vi "main.vi"() -> ()   [LabVIEW 2021]
uses:
  <vilib>/addons/Sound and Vibration/svt_Controls/subVIs/SV Intensity Graph.ctl
  <vilib>/sound2/lvsound2.llb/Sound Data Format.ctl
  <vilib>/sound2/lvsound2.llb/Sampling Mode.ctl
  <vilib>/Utility/error.llb/DialogType.ctl
  <vilib>/sound2/lvsound2.llb/Sound File Write Open.vi
  <vilib>/sound2/lvsound2.llb/Sound File Write (DBL).vi
  <vilib>/sound2/lvsound2.llb/Sound Input Read (DBL).vi
panel:
  in  "Tab Control":enum32{"Waveform", "STFT"}(tab)
  out "INPUT1":waveform(dbl)(graph)
  out "INPUT2":waveform(dbl)(graph)
  out "INPUT3":waveform(dbl)(graph)
  out "INPUT4":waveform(dbl)(graph)
  out "SV Intensity Graph 4":T1
  out "SV Intensity Graph 3":T1
  out "SV Intensity Graph":T1
  out "SV Intensity Graph 2":T1
  out "selected path":path
  in  "修改路径":bool=TRUE
  in  "sound format":T2={"sample rate (S/s)"=22050.0, "number of channels"=2, "bits per sample"=16}
  out "音频存储路径":path
  in  "开始录音":bool
  in  "Stop":bool=TRUE
  in  "关于东原":bool
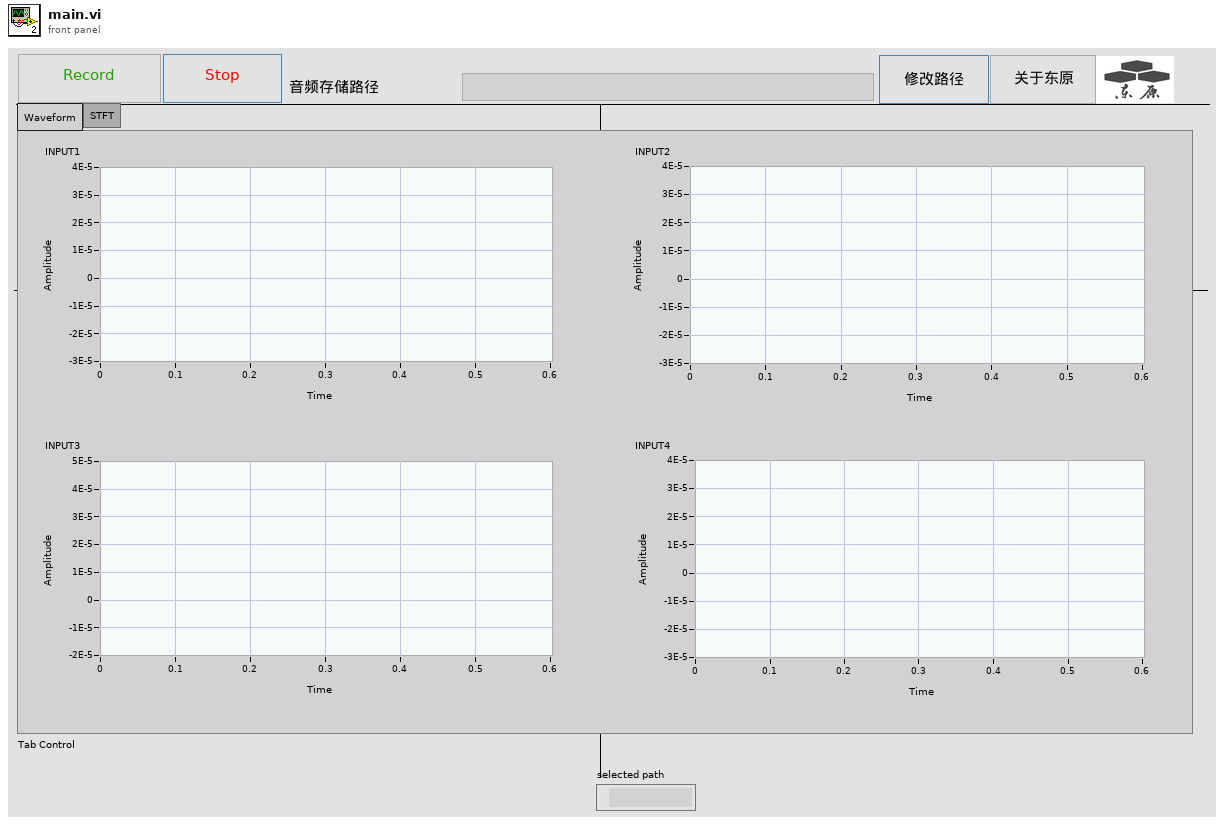
[diagram p1: front panel]
types:
  T1 = typedef "SV Intensity Graph.ctl" = dbl[][]
  T2 = typedef "Sound Data Format.ctl" = cluster{"sample rate (S/s)":dbl, "number of channels":i32, "bits per sample":i32}
  T3 = enum32{"invalid app kind", "Development System", "Run Time System", "Student Edition", "Embedded LabVIEW", "Evaluation", "Custom"}
  T4 = typedef "DialogType.ctl" = u16
  T5 = typedef "Sampling Mode.ctl" = i32
  T6 = typedef "Sound File Refnum.ctl" = refnum<file>
  T7 = typedef "Sound Input Task ID.ctl" = u32
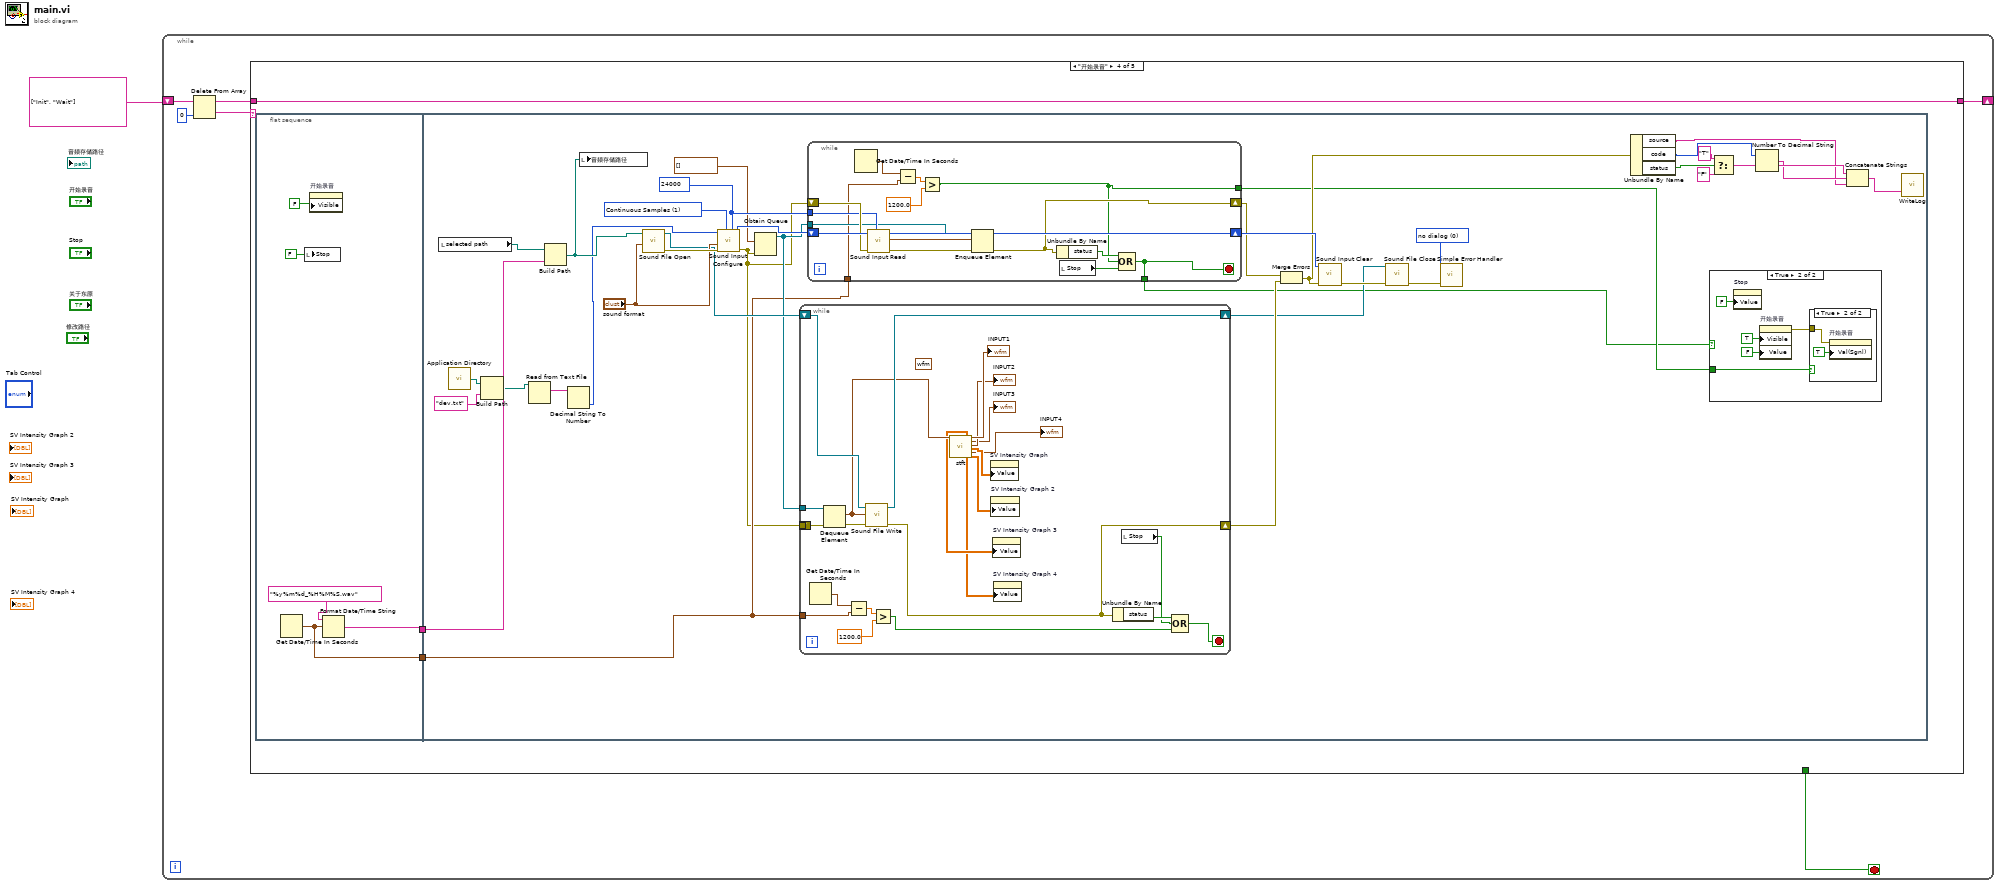
[diagram p0: block diagram]
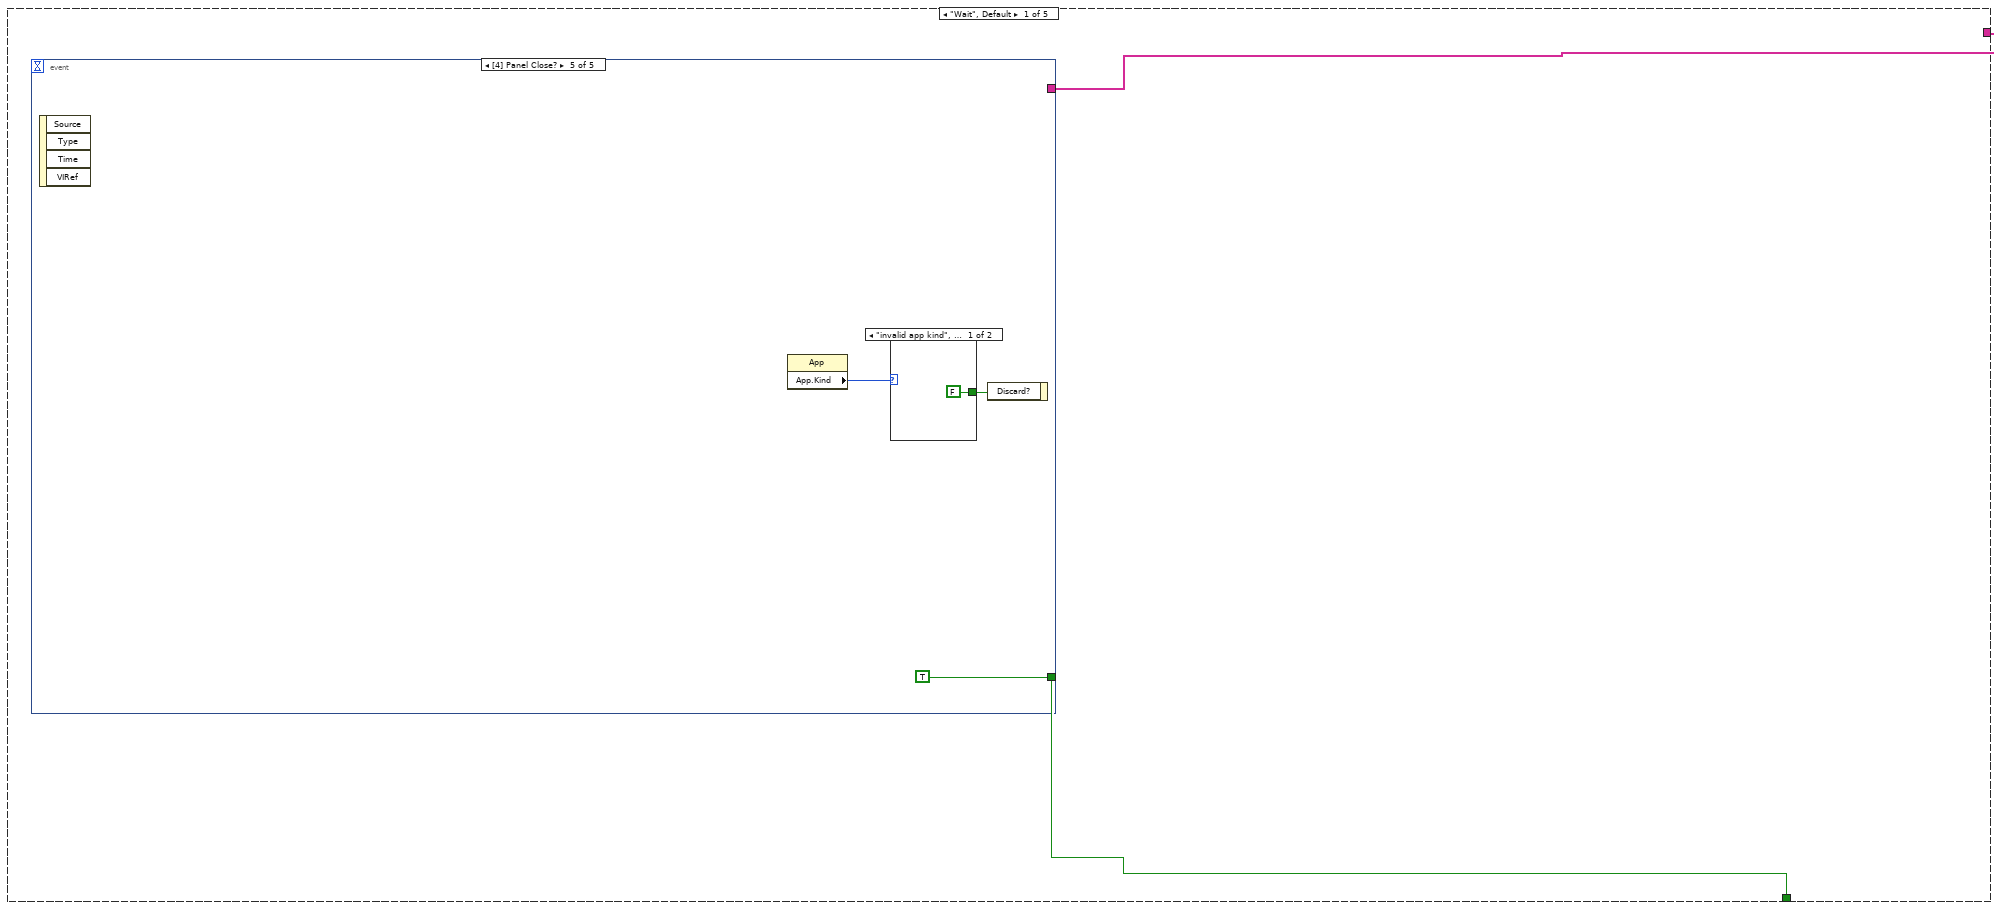
[diagram p2: hidden frame]
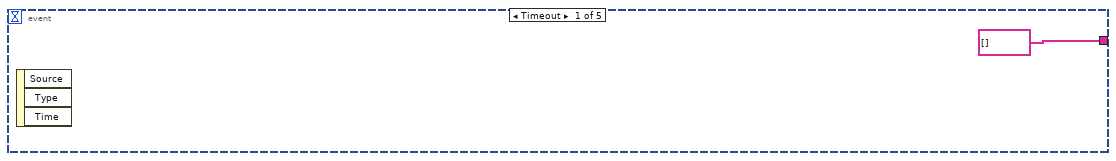
[diagram p3: hidden frame]
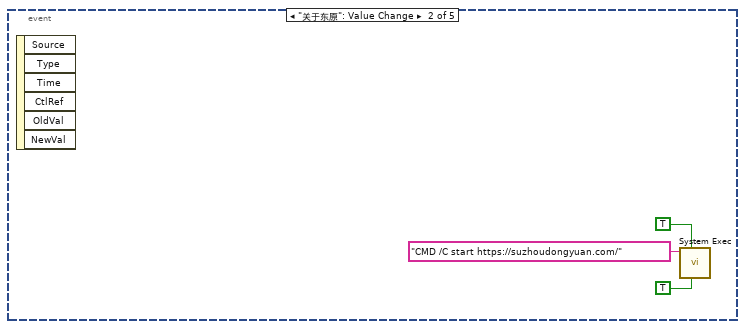
[diagram p4: hidden frame]
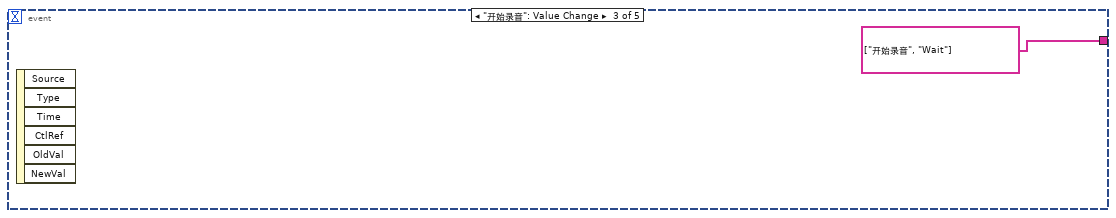
[diagram p5: hidden frame]
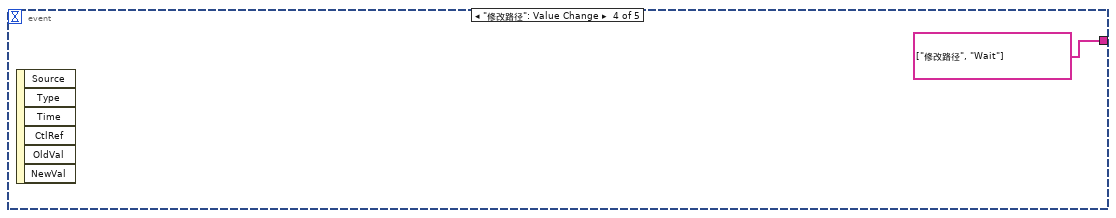
[diagram p6: hidden frame]
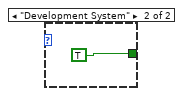
[diagram p7: hidden frame]
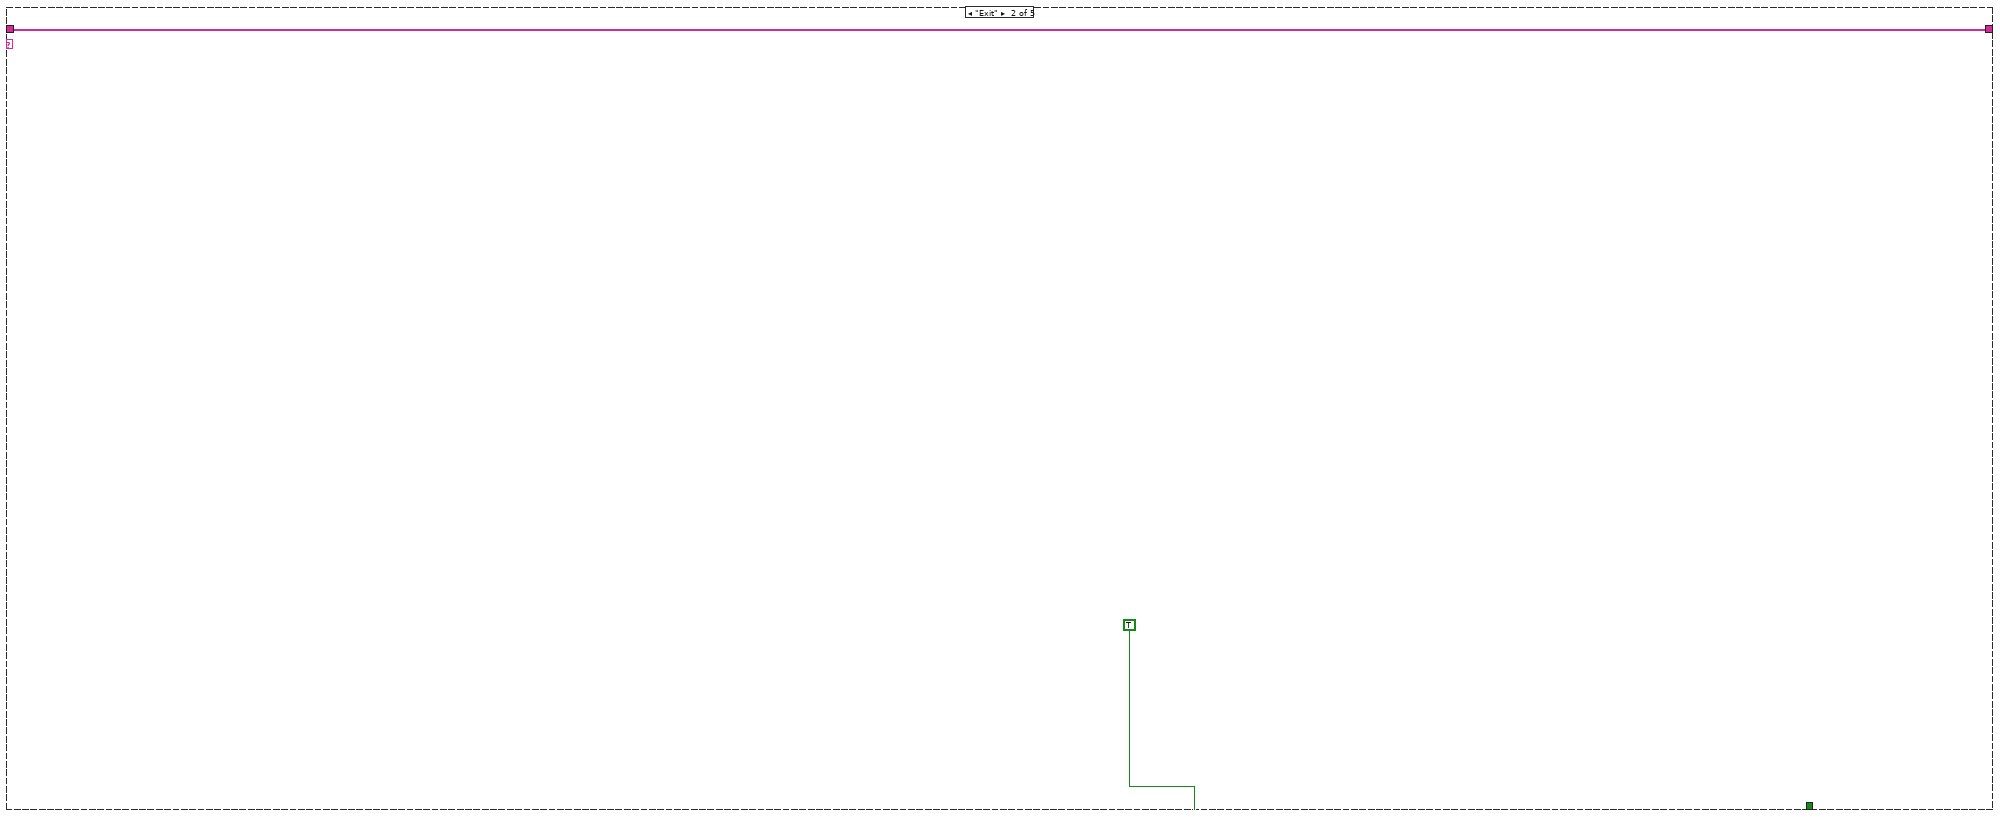
[diagram p8: hidden frame]
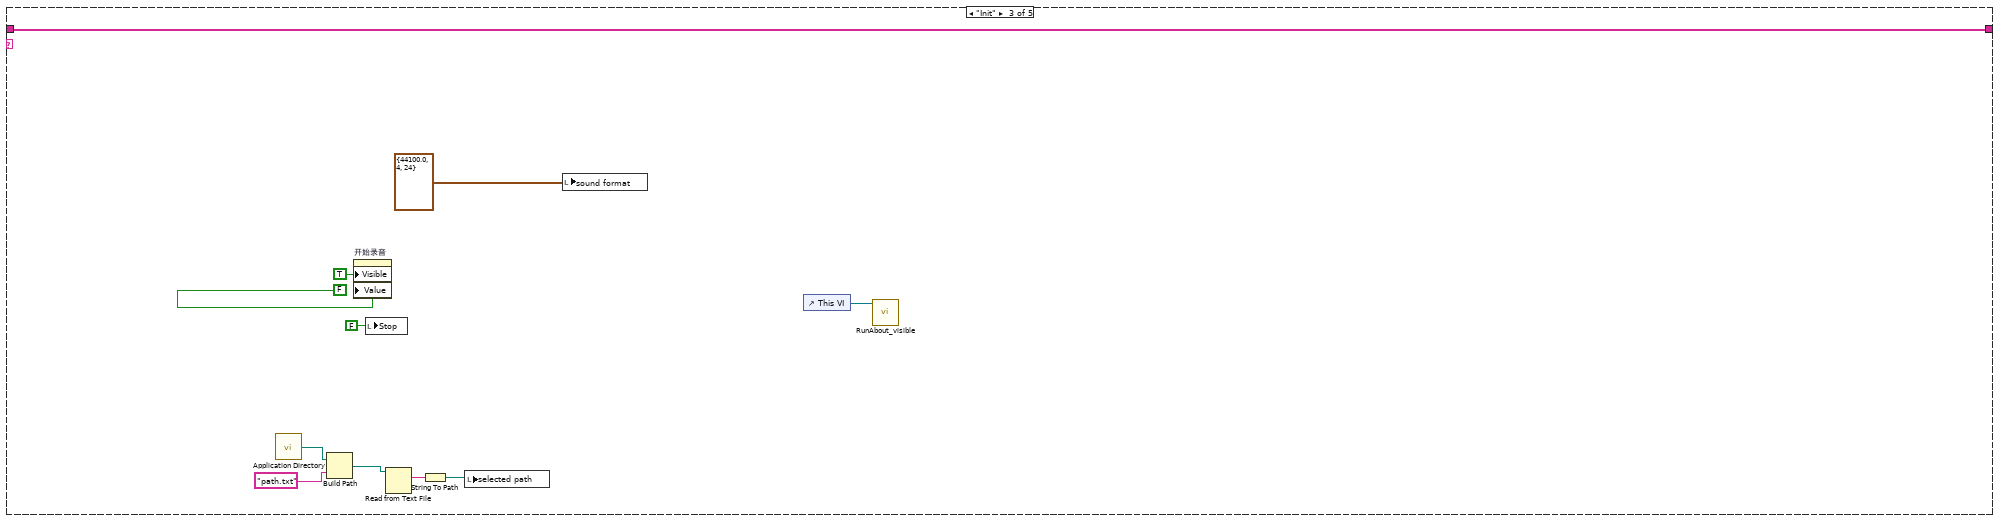
[diagram p9: hidden frame]
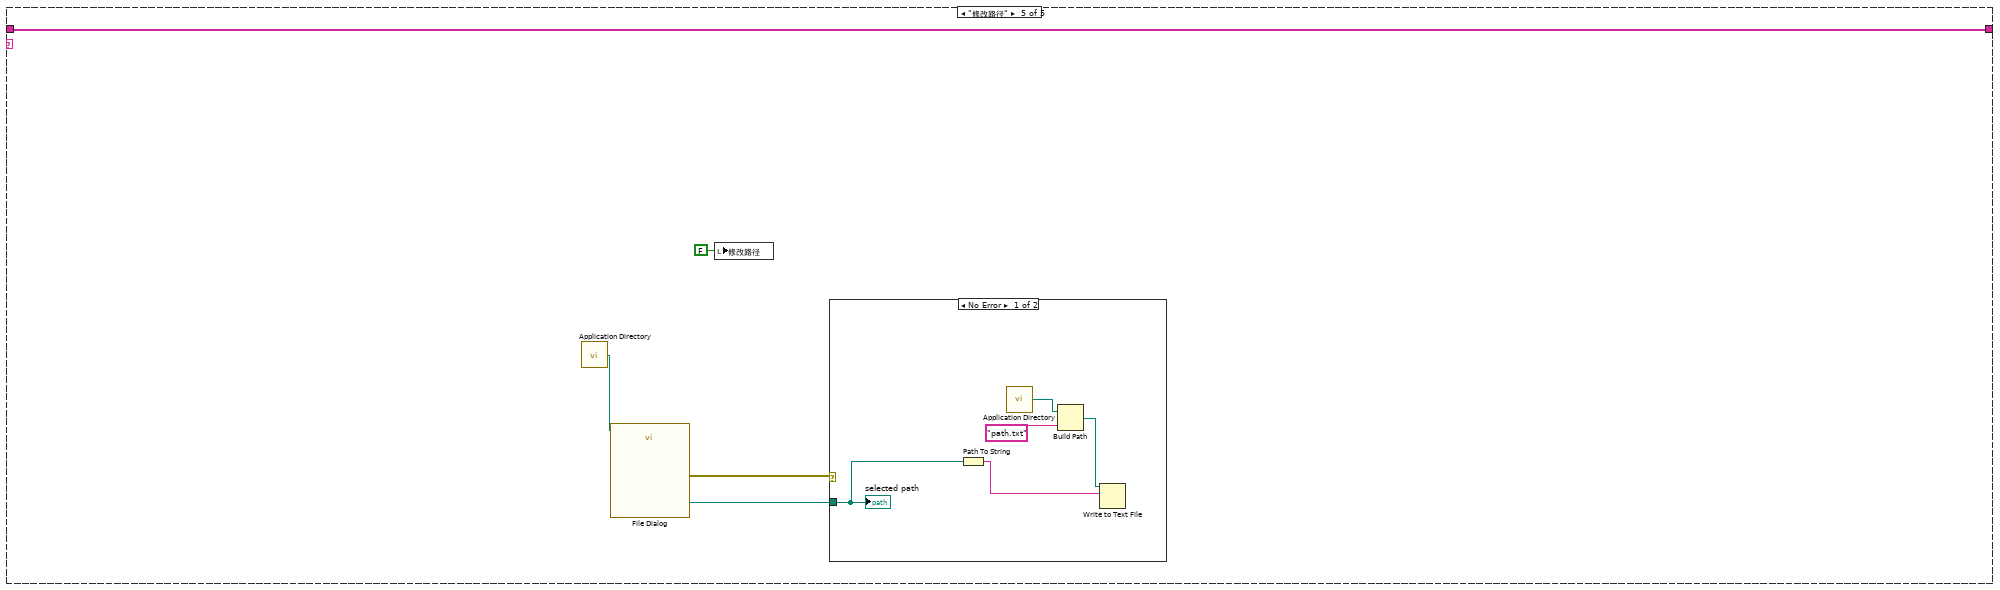
[diagram p12: hidden frame]
diagram:
  n1 = while {
    shift-right: [w3] -> _
    shift-left: string[] ["Init", "Wait"] -> [w7]
    stop <- w2 stop-if-true
    n2 = Delete From Array(array=w7, index=0 ("索引")) -> (deleted portion=w5:string, array with subset deleted=w4:string[])  [unwired: 1 in]
    n3 = case shown="\"开始录音\"" w5 {
      tunnel: w4 -> [_ w21 w33 w36 w128]
      tunnel: [w9 w21 w33 w36 w128] -> w3
      tunnel: [w8 TRUE _ _ _] -> w2
      frame "Wait", Default {
        n4 = event shown="[4] Panel Close?" {
          selector: _ -> [_ _ _ _ _]
          dyn-events: _ -> [_ _ _ _ _]
          timeout: _ -> [_ _ _ _ _]
          tunnel: [string[] [] _ string[] ["开始录音", "Wait"] string[] ["修改路径", "Wait"] _] -> w9
          tunnel: [_ _ _ _ TRUE] -> w8
          event Timeout {
            n5 = event-data() -> ()  [unwired: 1 in, 3 out]
          }
          event "关于东原": Value Change {
            n6 = event-data() -> ()  [unwired: 1 in, 6 out]
            n7 = call <vilib>:"System Exec.vi"("run minimized? (F)"=TRUE, "wait until completion? (T)"=TRUE, "command line"="CMD /C start https://suzhoudongyuan.com/") -> ()  [unwired: 5 in, 4 out]
          }
          event "开始录音": Value Change {
            n8 = event-data() -> ()  [unwired: 1 in, 6 out]
          }
          event "修改路径": Value Change {
            n9 = event-data() -> ()  [unwired: 1 in, 6 out]
          }
          event Panel Close? {
            n10 = event-data() -> ()  [unwired: 1 in, 4 out]
            n11 = property class="App"() -> ("App.Kind"=w18:T3)  [unwired: 2 in, 2 out]
            n12 = case shown="\"invalid app kind\", Default" w18 {
              tunnel: [FALSE ("放弃？") TRUE ("放弃？")] -> w17
              frame "invalid app kind", Default {
              }
              frame "Development System" {
              }
            }
            n13 = event-data("Discard?"=w17) -> ()  [unwired: 1 in, 1 out]
          }
        }
      }
      frame "Exit" {
      }
      frame "Init" {
        n14 = call <vilib>:"Application Directory.vi"() -> ("Application Directory"=w26:path)
        n15 = Build Path(base path=w26, name or relative path="path.txt") -> (appended path=w28:path)
        n16 = property on="开始录音" class="Bool (strict)"("Visible"=TRUE, "Value"=FALSE ("开始录音")) -> ()  [unwired: 2 in, 2 out]
        n17 = local write "Stop"(FALSE ("Stop")) -> ()
        n18 = Read from Text File(file (use dialog)=w28) -> (text=w29:string)  [unwired: 3 in, 3 out]
        n19 = String To Path(string=w29) -> (path=w25:path)
        n20 = local write "selected path"(w25) -> ()
        n21 = local write "sound format"(T2 {"sample rate (S/s)"=44100.0, "number of channels"=4, "bits per sample"=24} ("sound format")) -> ()
        n22 = control-ref of="This VI"() -> (w24:refnum<vi>)
        n23 = call "RunAbout_visible.vi"("This VI"=w24) -> ()  [unwired: 11 in]
      }
      frame "开始录音" {
        n24 = flat-sequence {
          tunnel: [w38] -> w35
          tunnel: [w37] -> w34
          tunnel: w35 -> [w77]
          tunnel: w34 -> [w58]
          frame #0 {
            n25 = Get Date/Time In Seconds() -> (seconds since 1Jan1904=w37:timestamp)
            n26 = local write "Stop"(FALSE ("Stop")) -> ()
            n27 = property on="开始录音" class="Bool (strict)"("Visible"=FALSE) -> ()  [unwired: 2 in, 2 out]
            n28 = Format Date/Time String(time format string (%c)="%y%m%d_%H%M%S.wav", seconds (now)=w37) -> (date/time string=w38:string)  [unwired: 1 in]
          }
          frame #1 {
            w71 = T4 0 items=["no dialog", "OK message", "continue or stop message", "OK message + warnings", "continue/stop + warnings"] ("type of dialog (OK msg:1)")
            w72 = 24000 ("number of samples/ch")
            w76 = T5 1 items=["Finite Samples", "Continuous Samples"] ("sample mode")
            n29 = local read "selected path"() -> (w47:path)
            n30 = call <vilib>:"Application Directory.vi"() -> ("Application Directory"=w43:path)
            n31 = Build Path(base path=w43, name or relative path="dev.txt") -> (appended path=w45:path)
            n32 = Read from Text File(file (use dialog)=w45) -> (text=w46:string)  [unwired: 3 in, 3 out]
            n33 = Build Path(base path=w47, name or relative path=w77) -> (appended path=w48:path)
            n34 = Decimal String To Number(string=w46) -> (number=w42:i32)  [unwired: 2 in, 1 out]
            n35 = local write "音频存储路径"(w48) -> ()
            n36 = call-poly <vilib>:"Sound File Open.vi"("sound format"="sound format", "path"=w48) -> ("error out"=w62:errorcluster, "sound file refnum"=w60:T6)  [unwired: 8 in]
            n37 = call <vilib>:"Sound Input Configure.vi"("number of samples/ch"=w72, "sample mode"=w76, "error in (no error)"=w62, "sound format"="sound format", "device ID"=w42) -> ("error out"=w57:errorcluster, "task ID"=w75:T7)  [unwired: 5 in]
            n38 = Obtain Queue(element data type=waveform(dbl)[] [] ("data"), error in (no error)=w57) -> (queue out=w59:refnum<queue>)  [unwired: 2 in, 3 out]
            n39 = while {
              shift-right: [w99] -> w52
              shift-left: w60 -> [w100]
              tunnel: w59 -> [w98]
              tunnel: w58 -> [w93]
              tunnel: w57 -> [w88]
              shift-right: [w86] -> w56
              shift-left: _ -> [_]
              stop <- w89 stop-if-true
              (unwired) waveform(dbl) {"t0"=timestamp(0 s since 1904-01-01), "dt"=1.0, "Y"=[]} ("INPUT3")
              n40 = Get Date/Time In Seconds() -> (seconds since 1Jan1904=w94:timestamp)
              n41 = Dequeue Element(queue=w98, error in (no error)=w88) -> (element=w97:waveform(dbl)[], error out=w87:errorcluster)  [unwired: 3 out]
              n42 = Subtract(x=w94, y=w93) -> (x-y=w91:dbl)
              n43 = call-poly <vilib>:"Sound File Write.vi"("error in (no error)"=w87, "data"=w97, "sound file refnum"=w100) -> ("error out"=w86:errorcluster, "sound file refnum out"=w99:T6)  [unwired: 7 in]
              n44 = Greater?(x=w91, y=1200.0) -> (0:w90:bool)
              n45 = call "stft.vi"("array"=w97) -> ("power spectra [dB EU] 3"=w79:dbl[][], "power spectra [dB EU] 4"=w78:dbl[][], "input1"=→"INPUT1":waveform(dbl), "input3"=→"INPUT3":waveform(dbl), "input2"=→"INPUT2":waveform(dbl), "power spectra [dB EU]"=w83:dbl[][], "input4"=→"INPUT4":waveform(dbl), "power spectra [dB EU] 2"=w82:dbl[][])  [unwired: 11 in]
              n46 = property on="SV Intensity Graph" class="IntGraph (strict)"("Value"=w83) -> ()  [unwired: 2 in, 2 out]
              n47 = property on="SV Intensity Graph 2" class="IntGraph (strict)"("Value"=w82) -> ()  [unwired: 2 in, 2 out]
              n48 = property on="SV Intensity Graph 3" class="IntGraph (strict)"("Value"=w79) -> ()  [unwired: 2 in, 2 out]
              n49 = property on="SV Intensity Graph 4" class="IntGraph (strict)"("Value"=w78) -> ()  [unwired: 2 in, 2 out]
              n50 = Unbundle By Name(w86) -> ("status"=w96:bool)
              n51 = local read "Stop"() -> (w95:bool)
              n52 = Compound Arithmetic op=OR(w96, w95, w90) -> (w89:bool)
            }
            n53 = while {
              tunnel: w72 -> [w113]
              shift-right: [w114] -> w74
              shift-left: w75 -> [w116]
              shift-right: [w110] -> w55
              shift-left: w57 -> [w115]
              tunnel: w59 -> [w112]
              tunnel: w58 -> [w105]
              tunnel: [w103] -> w50
              tunnel: [w102] -> w49
              stop <- w102 stop-if-true
              n54 = Get Date/Time In Seconds() -> (seconds since 1Jan1904=w106:timestamp)
              n55 = call-poly <vilib>:"Sound Input Read.vi"("number of samples/ch"=w113, "error in (no error)"=w115, "task ID"=w116) -> ("error out"=w111:errorcluster, "data"=w101:waveform(dbl)[], "task ID out"=w114:T7)  [unwired: 6 in]
              n56 = Subtract(x=w106, y=w105) -> (x-y=w108:dbl)
              n57 = Greater?(x=w108, y=1200.0) -> (0:w103:bool)
              n58 = Enqueue Element(queue=w112, element=w101, error in (no error)=w111) -> (error out=w110:errorcluster)  [unwired: 3 out]
              n59 = Unbundle By Name(w110) -> ("status"=w109:bool)
              n60 = local read "Stop"() -> (w104:bool)
              n61 = Compound Arithmetic op=OR(w109, w103, w104) -> (w102:bool)
            }
            n62 = Merge Errors(w55, w56) -> (w73:errorcluster)
            n63 = call <vilib>:"Sound Input Clear.vi"("error in (no error)"=w73, "task ID"=w74) -> ("error out"=w54:errorcluster)  [unwired: 9 in]
            n64 = call <vilib>:"Sound File Close.vi"("error in (no error)"=w54, "sound file refnum"=w52) -> ("error out"=w53:errorcluster)  [unwired: 9 in]
            n65 = call <vilib>:"Simple Error Handler.vi"("type of dialog (OK msg:1)"=w71, "error in (no error)"=w53) -> ()  [unwired: 3 in, 5 out]
            n66 = Unbundle By Name(w73) -> ("source"=w65:string, "code"=w67:i32, "status"=w51:bool)
            n67 = case shown="True" w49 {
              tunnel: w50 -> [_ w118]
              frame False {
              }
              frame True {
                n68 = property on="Stop" class="Bool (strict)"("Value"=FALSE ("Stop")) -> ()  [unwired: 2 in, 2 out]
                n69 = property on="开始录音" class="Bool (strict)"("Visible"=TRUE, "Value"=FALSE ("开始录音")) -> (error out=w117:errorcluster)  [unwired: 2 in, 1 out]
                n70 = case shown="True" w118 {
                  tunnel: w117 -> [_ w122]
                  frame False {
                  }
                  frame True {
                    n71 = property on="开始录音" class="Bool (strict)"(error in=w122, "Val(Sgnl)"=TRUE ("Value (Signaling)")) -> ()  [unwired: 1 in, 2 out]
                  }
                }
              }
            }
            n72 = Select(t="T", s=w51, f="F") -> (s? t:f=w68:string)
            n73 = Number To Decimal String(number=w67) -> (decimal integer string=w66:string)  [unwired: 1 in]
            n74 = Concatenate Strings(w68, w66, w65) -> (w64:string)
            n75 = call "WriteLog.vi"("String"=w64) -> ()  [unwired: 2 in]
          }
        }
      }
      frame "修改路径" {
        n76 = call <vilib>:"Application Directory.vi"() -> ("Application Directory"=w127:path)
        n77 = call "File Dialog"("start path"=w127) -> ("selected path"=w125:path, "error out"=w126:errorcluster)  [unwired: 11 in, 2 out]
        n78 = local write "修改路径"(FALSE ("修改路径")) -> ()
        n79 = case shown="No Error" w126 {
          tunnel: w125 -> [w129 _]
          frame No Error {
            n80 = Path To String(path=w129) -> (string=w130:string)
            n81 = call <vilib>:"Application Directory.vi"() -> ("Application Directory"=w131:path)
            n82 = Build Path(base path=w131, name or relative path="path.txt") -> (appended path=w133:path)
            n83 = Write to Text File(file (use dialog)=w133, text=w130) -> ()  [unwired: 2 in, 3 out]
            "selected path" <- w129
          }
          frame Error {
          }
        }
      }
    }
  }
